vi "Agilent SNA Set External Trigger Mode.vi"(4 "Passthrough (T)":bool=TRUE, 7 "Agilent SNA & SWP":T1, 8 "error in (no error)":errorcluster, 10 "Ext. Trigger Mode":T2, 11 "VISA Resource Names":T3) -> (0 "error out":errorcluster, 3 "dup VISA Resource Names":T3)   [LabVIEW 2011]
doc: "This VI for the HP8753B Network Analyzers reads the stimulus values. Except when performing log sweeps and freq list sweeps, this VI uses the start and stop values and the number of points to calcuate the stimulus values."
uses:
  TypeDefs/Agilent SNA VISA.ctl
  TypeDefs/Agilent SNA External Trigger Mode.ctl
  TypeDefs/Agilent SNA Instrument Info.ctl
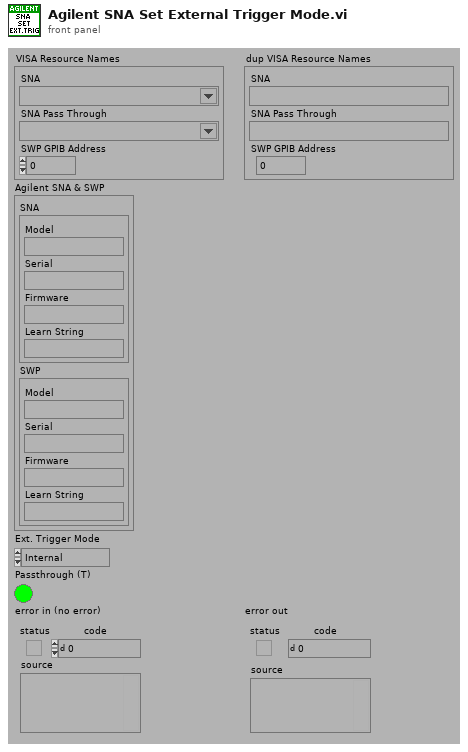
[diagram p1: front panel]
types:
  T1 = typedef "Agilent SNA Instrument Info.ctl" = cluster{"SNA":cluster{"Model":string, "Serial":string, "Firmware":string, "Learn String":string}, "SWP":cluster{"Model":string, "Serial":string, "Firmware":string, "Learn String":string}}
  T2 = typedef "Agilent SNA External Trigger Mode.ctl" = enum16{"Internal", "External", "Single/Bus"}
  T3 = typedef "Agilent SNA VISA.ctl" = cluster{"SNA":refnum<visa-resource-name>, "SNA Pass Through":refnum<visa-resource-name>, "SWP GPIB Address":i32}
  T4 = typedef "Agilent SNA Model.ctl" = enum16{"Not Supported", "8757X"}
  T5 = typedef "Agilent SNA SWP Model.ctl" = enum16{"Not Supported", "836XXX", "8375XX", "E82X7D"}
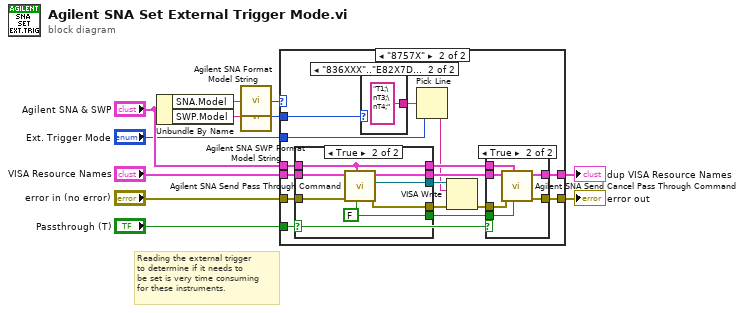
[diagram p0: block diagram]
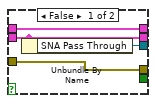
[diagram p4: hidden frame]
diagram:
  # "Reading the external trigger\nto determine if it needs to\nbe set is very time consuming\nfor these instruments."
  n1 = Unbundle By Name("Agilent SNA & SWP") -> ("SNA.Model"=w10:string, "SWP.Model"=w7:string)
  n2 = call "Agilent SNA Format Model String.vi"("Model String"=w10) -> ("Model"=w9:T4)
  n3 = call "Agilent SNA SWP Format Model String.vi"("Model String"=w7) -> ("Model"=w6:T5)
  n4 = case shown="\"8757X\"" w9 {
    tunnel: [w13 w20] -> w11
    tunnel: "Ext. Trigger Mode" -> [_ w29]
    tunnel: "error in (no error)" -> [w13 w19]
    tunnel: "VISA Resource Names" -> [w12 w18]
    tunnel: "Agilent SNA & SWP" -> [_ w17]
    tunnel: w6 -> [_ w27]
    tunnel: [w12 w15] -> w2
    tunnel: "Passthrough (T)" -> [_ w14]
    frame "Not Supported" {
    }
    frame "8757X" {
      n5 = case shown="True" w14 {
        tunnel: [w39 w48] -> w25
        tunnel: w19 -> [w40 w47]
        tunnel: w18 -> [w38 w46]
        tunnel: [w40 w45] -> w23
        tunnel: w17 -> [w41 w42]
        tunnel: [w38 w44] -> w22
        tunnel: [_ w43] -> w26
        tunnel: [w41 w42] -> w21
        frame False {
          n6 = Unbundle By Name(w38) -> ("SNA Pass Through"=w39:refnum<visa-resource-name>)
        }
        frame True {
          w43 = FALSE ("SCPI? (F)")
          n7 = call "Agilent SNA Send Pass Through Command.vi"("SCPI? (F)"=w43, "Agilent SNA & SWP"=w42, "error in (no error)"=w47, "VISA Resource Names"=w46) -> ("error out"=w45:errorcluster, "SNA Pass Through"=w48:refnum<visa-resource-name>, "dup VISA Resource Names"=w44:T3)  [unwired: 5 out]
        }
      }
      n8 = case shown="\"836XXX\"..\"E82X7D\"" w27 {
        tunnel: [_ "T1;\nT3;\nT4;"] -> w28
        frame "Not Supported" {
        }
        frame "836XXX".."E82X7D" {
        }
      }
      n9 = Pick Line(multi-line string=w28, line index=w29) -> (output string=w16:string)  [unwired: 1 out]
      n10 = VISA Write(VISA resource name=w25, write buffer=w16, error in (no error)=w23) -> (error out=w24:errorcluster)  [unwired: 2 out]
      n11 = case shown="True" w14 {
        tunnel: [w31 w37] -> w20
        tunnel: w22 -> [w30 w36]
        tunnel: w24 -> [w31 w35]
        tunnel: w26 -> [_ w34]
        tunnel: [w30 w33] -> w15
        tunnel: w21 -> [_ w32]
        frame False {
        }
        frame True {
          n12 = call "Agilent SNA Send Cancel Pass Through Command.vi"("SCPI? (F)"=w34, "Agilent SNA & SWP"=w32, "error in (no error)"=w35, "VISA Resource Names"=w36) -> ("error out"=w37:errorcluster, "dup VISA Resource Names"=w33:T3)  [unwired: 6 out]
        }
      }
    }
  }
  "dup VISA Resource Names" <- w2
  "error out" <- w11
